vi "Set Selector test.vi"(8 "error in (no error)":errorcluster caption="entrée d'erreur (pas d'erreur)", 10 "Selector test":cluster{"Booléen 4":bool}[](array[cluster])=[{"Booléen 4"=TRUE}, {"Booléen 4"=TRUE}, {"Booléen 4"=TRUE}, {"Booléen 4"=TRUE}, {"Booléen 4"=TRUE}, {"Booléen 4"=TRUE}, {"Booléen 4"=TRUE}, {"Booléen 4"=TRUE}], 11 "Sequencer (Default) en entrée":refnum<class "Sequencer (Default).lvclass">) -> (0 "error out":errorcluster caption="sortie d'erreur", 3 "Sequencer (Default) en sortie":refnum<class "Sequencer (Default).lvclass">)   [LabVIEW 2020, in "Library Core.lvlib" / "Sequencer (Default).lvclass"]
uses:
  Sequencer (Default).lvclass
  Sequencer (Default).lvclass/Sequencer (Default).ctl
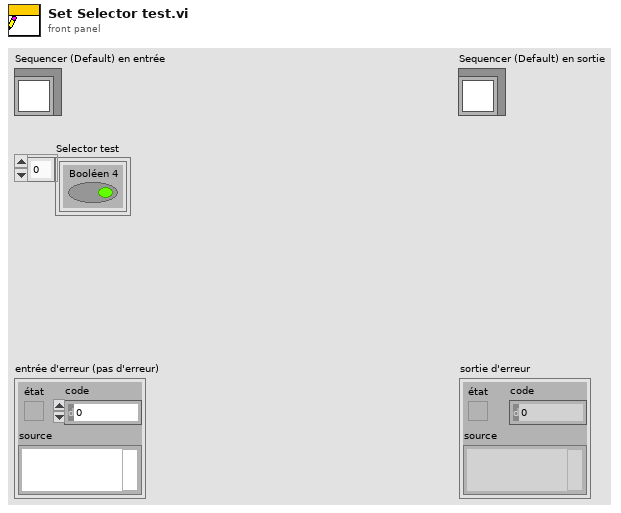
[diagram p1: front panel]
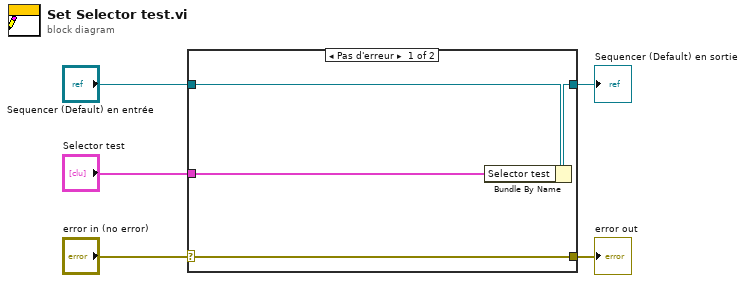
[diagram p0: block diagram]
diagram:
  n1 = case shown="Pas d'erreur" "error in (no error)" {
    selector: "error in (no error)" -> [w9 w10]
    tunnel: [w9 w10] -> w4
    tunnel: [w7 w11] -> w2
    tunnel: "Sequencer (Default) en entrée" -> [w8 w11]
    tunnel: "Selector test" -> [w6 _]
    frame No Error {
      n2 = Bundle By Name(cluster=w8, "Selector test"=w6) -> (w7:refnum<class "Sequencer (Default).lvclass">)
    }
    frame Error {
    }
  }
  "error out" <- w4
  "Sequencer (Default) en sortie" <- w2
